vi "Util_Convert String to Hex String.vi"(4 "Input String":string caption="Input HEX Description String") -> (1 "Output String":string caption="Output HEX String")   [LabVIEW 2014]
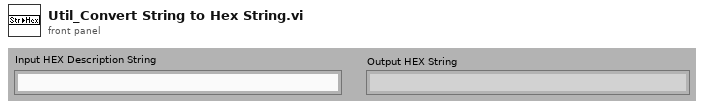
[diagram p1: front panel]
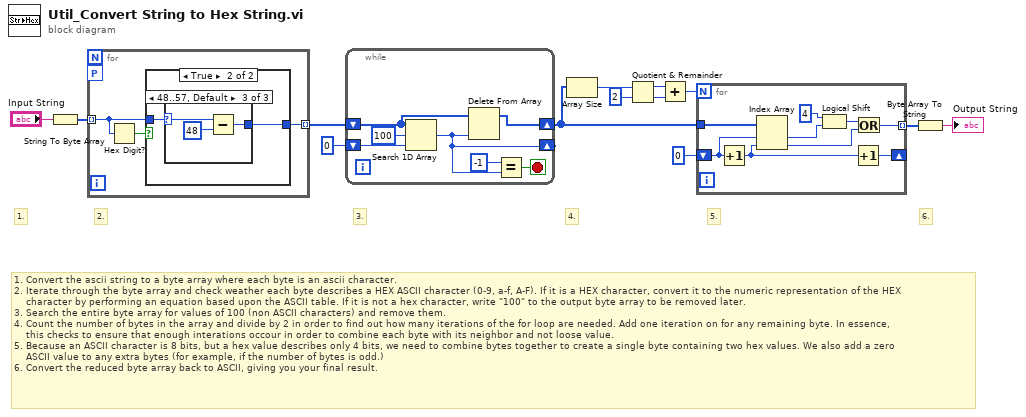
[diagram p0: block diagram]
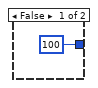
[diagram p2: hidden frame]
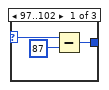
[diagram p3: hidden frame]
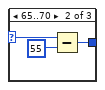
[diagram p4: hidden frame]
diagram:
  # "1. Convert the ascii string to a byte array where each byte is an ascii character.\n2. Iterate through the byte array and check weather each byte describes a HEX ASCII character (0-9, a-f, A-F). If it is a HEX character, convert it to the numeric representation of the HEX\n    character by performing an equation based upon the ASCII table. If it is not a hex character, write \"100\" to the output byte array to be removed later.\n3. Search the entire byte array for values of 100 (non ASCII characters) and remove them.\n4. Count the number of bytes in the array and divide by 2 in order to find out how many iterations of the for loop are needed. Add one iteration on for any remaining byte. In essence,\n    this checks to ensure that enough interations occour in order to combine each byte with its neighbor and not loose value.\n5. Because an ASCII character is 8 bits, but a hex value describes only 4 bits, we need to combine bytes together to create a single byte containing two hex values. We also add a zero\n    ASCII value to any extra bytes (for example, if the number of bytes is odd.)\n6. Convert the reduced byte array back to ASCII, giving you your final result."
  # "6."
  # "5."
  # "4."
  # "3."
  # "2."
  # "1."
  n1 = String To Byte Array(string="Input String") -> (unsigned byte array=w13:u8[])
  n2 = for {
    tunnel: w13 -> [w15] mode=indexing
    tunnel: [w14] -> w12 mode=indexing
    workers-P: _ -> [_]
    n3 = Hex Digit?(1:w15) -> (0:w16:bool)
    n4 = case shown="True" w16 {
      tunnel: w15 -> [_ w19]
      tunnel: [u8 100 w18] -> w14
      frame False {
      }
      frame True {
        n5 = case shown="48..57, Default" w19 {
          selector: w19 -> [w21 w23 w26]
          tunnel: [w22 w25 w28] -> w18
          frame 97..102 {
            n6 = Subtract(x=w21, y=u8 87 ("x")) -> (x-y=w22:u8)
          }
          frame 65..70 {
            n7 = Subtract(x=w23, y=u8 55 ("x")) -> (x-y=w25:u8)
          }
          frame 48..57, Default {
            n8 = Subtract(x=w26, y=u8 48 ("x")) -> (x-y=w28:u8)
          }
        }
      }
    }
  }
  n9 = while {
    shift-right: [w31] -> w9
    shift-left: w12 -> [w32]
    shift-right: [w30] -> _
    shift-left: 0 ("index of element") -> [w29]
    stop <- w33 stop-if-true
    n10 = Search 1D Array(1D array=w32, element=u8 100, start index (0)=w29) -> (index of element=w30:i32)
    n11 = Delete From Array(array=w32, index=w30) -> (array with subset deleted=w31:u8[])  [unwired: 1 in, 1 out]
    n12 = Equal?(x=-1, y=w30) -> (x = y?=w33:bool)
  }
  n13 = Array Size(array=w9) -> (size(s)=w8:i32)
  n14 = Quotient & Remainder(x=w8, y=2) -> (x-y*floor(x/y)=w5:i32, floor(x/y)=w6:i32)
  n15 = Add(x=w5, y=w6) -> (x+y=w4:i32)
  n16 = for {
    N: w4 -> [_]
    tunnel: w9 -> [w44]
    shift-right: [w42] -> _
    shift-left: 0 ("index") -> [w43]
    tunnel: [w39] -> w3 mode=indexing
    n17 = Increment(x=w43) -> (x+1=w41:i32)
    n18 = Index Array(array=w44, index #1=w43, index #2=w41) -> (element #1=w38:u8, element #2=w36:u8)
    n19 = Logical Shift(y=i8 4, x=w38) -> (x << y=w37:u8)
    n20 = Increment(x=w41) -> (x+1=w42:i32)
    n21 = Or(x=w37, y=w36) -> (x .or. y?=w39:u8)
  }
  n22 = Byte Array To String(unsigned byte array=w3) -> (string=→"Output String":string)
